vi "CRYSet One Quick Lunch Menu Front Panel.vi"(11 "Vi Ref In":refnum<vi> caption="Vi Ref") -> (3 "Vi Ref Out":refnum<vi> caption="Vi Ref")   [LabVIEW 2013]
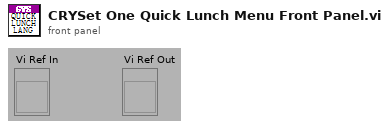
[diagram p1: front panel]
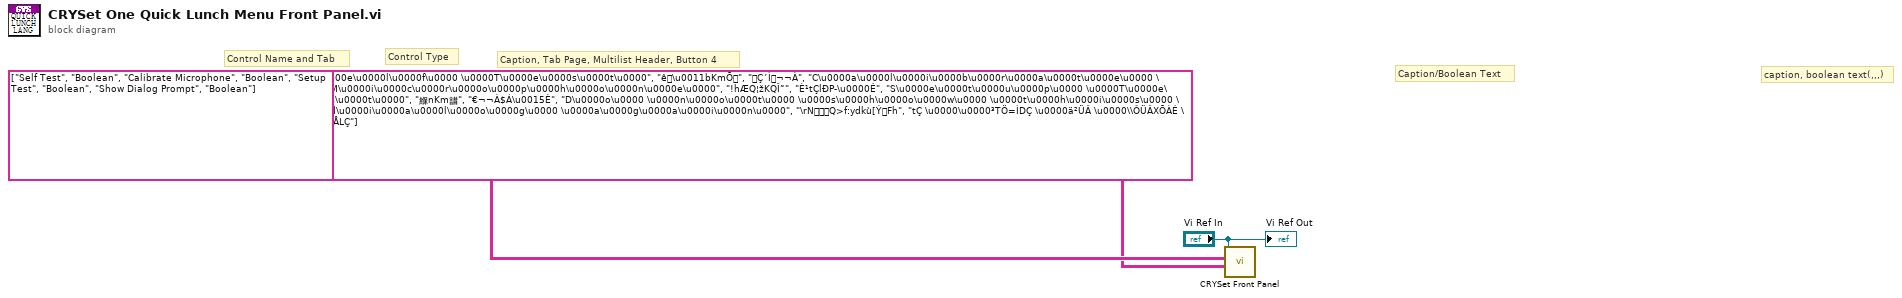
[diagram p0: block diagram]
diagram:
  # "Caption, Tab Page, Multilist Header, Button 4"
  # "Control Type"
  # "Control Name and Tab"
  # "caption, boolean text(,,,)"
  # "Caption/Boolean Text"
  n1 = call "CRYSet Front Panel.vi"("Caption(Boolean Text)"=string[][] [["S\u0000e\u0000l\u0000f\u0000 \u0000T\u0000e\u0000s\u0000t\u0000", "ê\u0011bKmÕ", "Ç´Ì¬¬À"], ["C\u0000a\u0000l\u0000i\u0000b\u0000r\u0000a\u0000t\u0000e\u0000 \u0000M\u0000i\u0000c\u0000r\u0000o\u0000p\u0000h\u0000o\u0000n\u0000e\u0000", "!hÆQ¦žKQÎ˜", "È¹tÇlÐP­\u0000É"], ["S\u0000e\u0000t\u0000u\u0000p\u0000 \u0000T\u0000e\u0000s\u0000t\u0000", "緥nKm諎", "€¬¬À$Á\u0015È"], ["D\u0000o\u0000 \u0000n\u0000o\u0000t\u0000 \u0000s\u0000h\u0000o\u0000w\u0000 \u0000t\u0000h\u0000i\u0000s\u0000 \u0000d\u0000i\u0000a\u0000l\u0000o\u0000g\u0000 \u0000a\u0000g\u0000a\u0000i\u0000n\u0000", "\rNQ>f:ydkù[ÝFh", "tÇ \u0000\u0000³TÖ=ÌDÇ \u0000ä²ÜÂ \u0000\\ÔÜÂXÕÀÉ \u0000JÅLÇ"]], "Control ID and Type(Label Name, Type)"=string[][] [["Self Test", "Boolean"], ["Calibrate Microphone", "Boolean"], ["Setup Test", "Boolean"], ["Show Dialog Prompt", "Boolean"]], "Vi Ref"="Vi Ref In") -> ()  [unwired: 9 in]
  "Vi Ref Out" <- "Vi Ref In"
